vi "Write Guidance Cluster.vi"(8 "error in (no error)":errorcluster, 10 "Guidance Cluster":T1={"Set Origin"=TRUE, "New WP"=FALSE, "Types of Change"=enum."Current NED", "Make Change"=FALSE, "Optimal Heading"=FALSE, "New SetPoint"={"North"=0.0, "East"=0.0, "Depth"=0.0, "Heading"=0.0}, "Update Reference"={"Mode Change"=FALSE, "Current Position"=[]}, "Go"=FALSE, "Go heading"=FALSE}, 11 "Supervisor in":refnum<class "Supervisor.lvclass">) -> (0 "error out":errorcluster, 3 "Supervisor out":refnum<class "Supervisor.lvclass">)   [LabVIEW 2014, in "Supervisor.lvclass"]
uses:
  Supervisor.lvclass
  Supervisor.lvclass/Supervisor.ctl
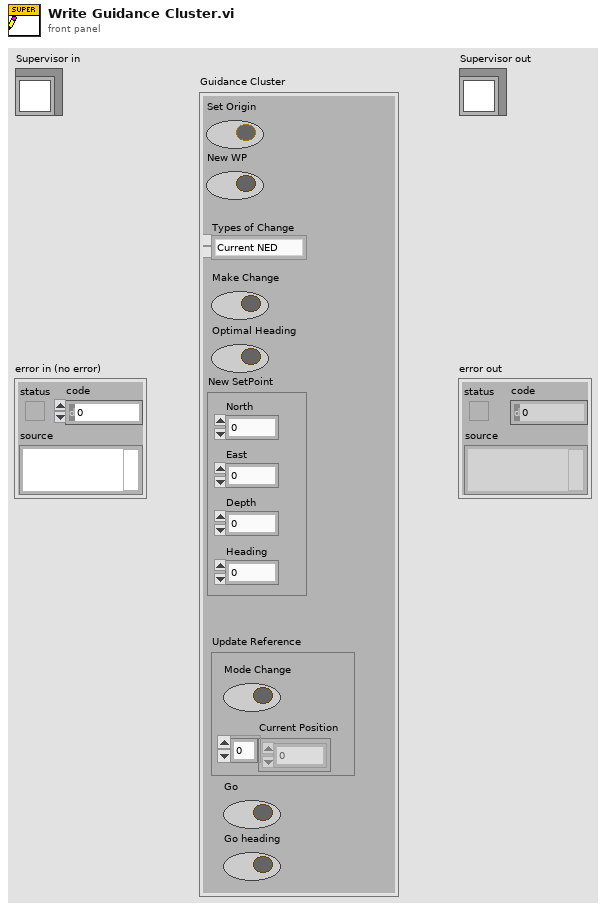
[diagram p1: front panel]
types:
  T1 = cluster{"Set Origin":bool, "New WP":bool, "Types of Change":enum16{"Current NED", "Change NED"}, "Make Change":bool, "Optimal Heading":bool, "New SetPoint":cluster{"North":dbl, "East":dbl, "Depth":dbl, "Heading":dbl}, "Update Reference":cluster{"Mode Change":bool, "Current Position":dbl[]}, "Go":bool, "Go heading":bool}
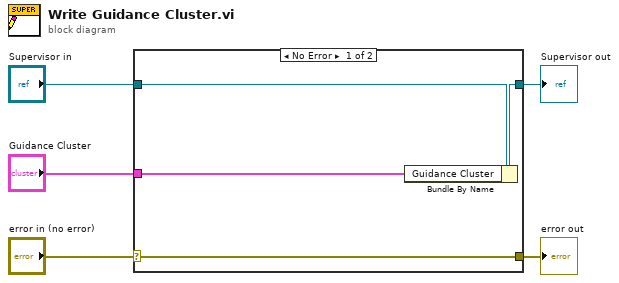
[diagram p0: block diagram]
diagram:
  n1 = case shown="No Error" "error in (no error)" {
    selector: "error in (no error)" -> [w9 w10]
    tunnel: [w9 w10] -> w4
    tunnel: [w7 w11] -> w2
    tunnel: "Supervisor in" -> [w8 w11]
    tunnel: "Guidance Cluster" -> [w6 _]
    frame No Error {
      n2 = Bundle By Name(cluster=w8, "Guidance Cluster"=w6) -> (w7:refnum<class "Supervisor.lvclass">)
    }
    frame Error {
    }
  }
  "error out" <- w4
  "Supervisor out" <- w2
